vi "Subpanel Plugin Connect Event.vi"(8 "error in (no error)":errorcluster, 10 "Address and Port":string, 11 "CIF_UI in":refnum<class "CIF_UI.lvclass">) -> (0 "error out":errorcluster)   [LabVIEW 2021, in "CIF_UI.lvclass"]
uses:
  CIF_UI.lvclass
  CIF_UI.lvclass/CIF_UI.ctl
  Typedef/New Connection Plugin Event Data.ctl
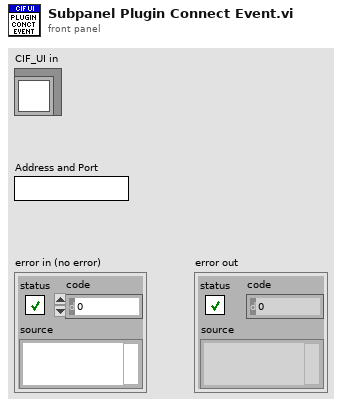
[diagram p1: front panel]
types:
  T1 = typedef "CIF_UI.lvclass/New Connection Plugin Event Data.ctl" = cluster{"IP Address and Port":string, "Connected":bool}
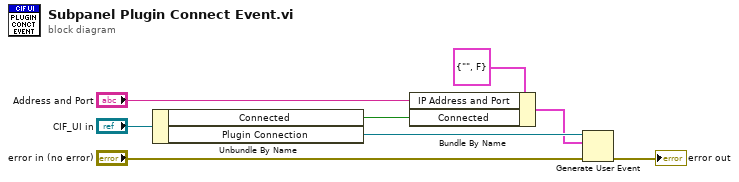
[diagram p0: block diagram]
diagram:
  n1 = Unbundle By Name("CIF_UI in") -> ("Connected"=w4:bool, "Plugin Connection"=w5:refnum<user-event>)
  n2 = Bundle By Name(cluster=T1 {"IP Address and Port"="", "Connected"=FALSE} ("event data"), "IP Address and Port"="Address and Port", "Connected"=w4) -> (w1:T1)
  n3 = Generate User Event(user event=w5, event data cluster=w1, error in="error in (no error)") -> (error out=→"error out":errorcluster)  [unwired: 1 in, 1 out]
